vi "Array Comparison.vi"(1 "Bit STream 2":i32[](array[numeric]) caption="bit stream 2", 2 "Bit Stream 1":i32[](array[numeric]) caption="bit stream 1") -> (0 "Bit Stream Comparison":bool[](array[boolean]))   [LabVIEW 2018]
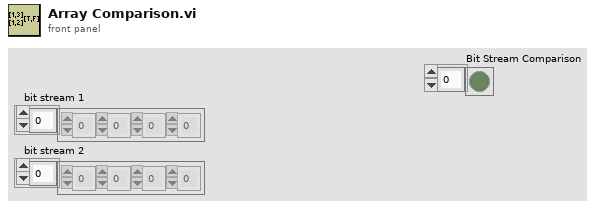
[diagram p1: front panel]
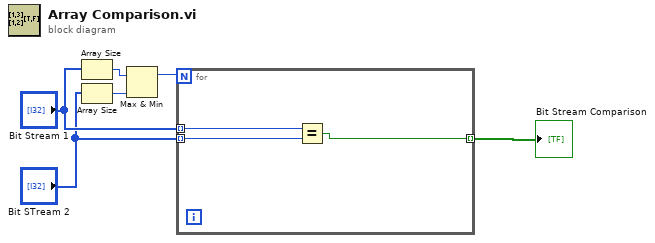
[diagram p0: block diagram]
diagram:
  n1 = Array Size(array="Bit Stream 1") -> (size(s)=w5:i32)
  n2 = Array Size(array="Bit STream 2") -> (size(s)=w4:i32)
  n3 = Max & Min(x=w5, y=w4) -> (max(x,y)=w6:i32)  [unwired: 1 out]
  n4 = for {
    N: w6 -> [_]
    tunnel: "Bit Stream 1" -> [w9] mode=indexing
    tunnel: "Bit STream 2" -> [w8] mode=indexing
    tunnel: [w7] -> w1 mode=indexing
    n5 = Equal?(x=w9, y=w8) -> (x = y?=w7:bool)
  }
  "Bit Stream Comparison" <- w1
